vi "Str To UTF16.vi"(1 "String":string) -> (0 "WideString (UTF16)":string)   [LabVIEW 2012]
doc: "Converts a standard ASCII string to UTF16."
uses:
  kernel32.dll
panel:
  out "error out":errorcluster
  in  "error in (no error)":errorcluster
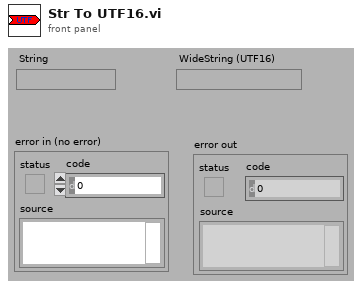
[diagram p1: front panel]
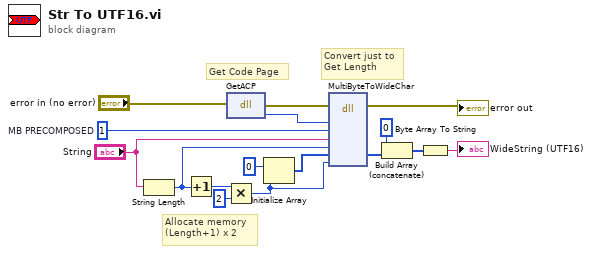
[diagram p0: block diagram]
diagram:
  w16 = u32 1  # MB PRECOMPOSED
  # "Convert just to\nGet Length"
  # "Get Code Page"
  # "Allocate memory\n(Length+1) x 2"
  n1 = String Length(string="String") -> (length=w1:i32)
  n2 = Increment(x=w1) -> (x+1=w4:i32)
  n3 = Multiply(x=w4, y=2) -> (x*y=w2:i32)
  n4 = dll-call lib="kernel32.dll" fn="GetACP" ("GetACP()")(error in="error in (no error)") -> (error out=w14:errorcluster, w15:u32)  [unwired: 2 in, 1 out]
  n5 = Initialize Array(u16 0, w2) -> (w6:u16[])
  n6 = dll-call lib="kernel32.dll" fn="MultiByteToWideChar"(error in=w14, "codePage"=w15, "dwFlags"=w16, "lpCStr"="String", "nChars"=w1, "lpWStr"=w6, "nWStr"=w2) -> (error out=→"error out":errorcluster, "lpWStr"=w10:u8[])  [unwired: 7 in, 2 out]
  n7 = Build Array (concatenate)(u16 0, w10) -> (w8:u16[])
  n8 = Byte Array To String(unsigned byte array=w8) -> (string=→"WideString (UTF16)":string)
